vi "Open Recording File.vi"(8 "error in (no error)":errorcluster, 11 "IntanElectrophysiology in":refnum<class "IntanElectrophysiology.lvclass">) -> (0 "error out":errorcluster, 3 "IntanElectrophysiology out":refnum<class "IntanElectrophysiology.lvclass">)   [LabVIEW 2014, in "IntanElectrophysiology.lvclass"]
uses:
  IntanElectrophysiology.lvclass
  IntanElectrophysiology.lvclass/IntanElectrophysiology.ctl
  AcquireTraces/AcquireTraces.lvclass/AcquireTraces.ctl
  HDF5Tools/LabView/Create Dataset 2D Integer.vi
  HDF5Tools/LabView/HDF5Tools.lvlib
  AcquireTraces/AcquireTraces.lvclass
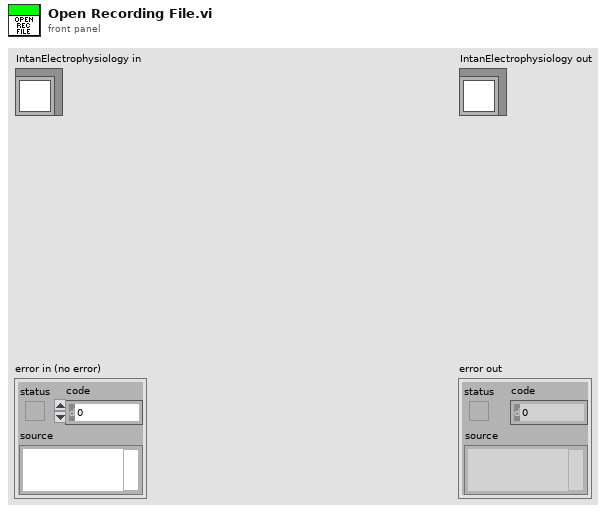
[diagram p1: front panel]
types:
  T1 = cluster{"Channels":string[], "SampClkRate":dbl, "AIDevScalingCoeff":dbl[], "Acq Channel Number":i32[], "Num Preamp Streams":i32, "Chans Per Preamp Stream":i32, "Num Board Channels":i32, "Samples Per Pkt Per Chan":i32}
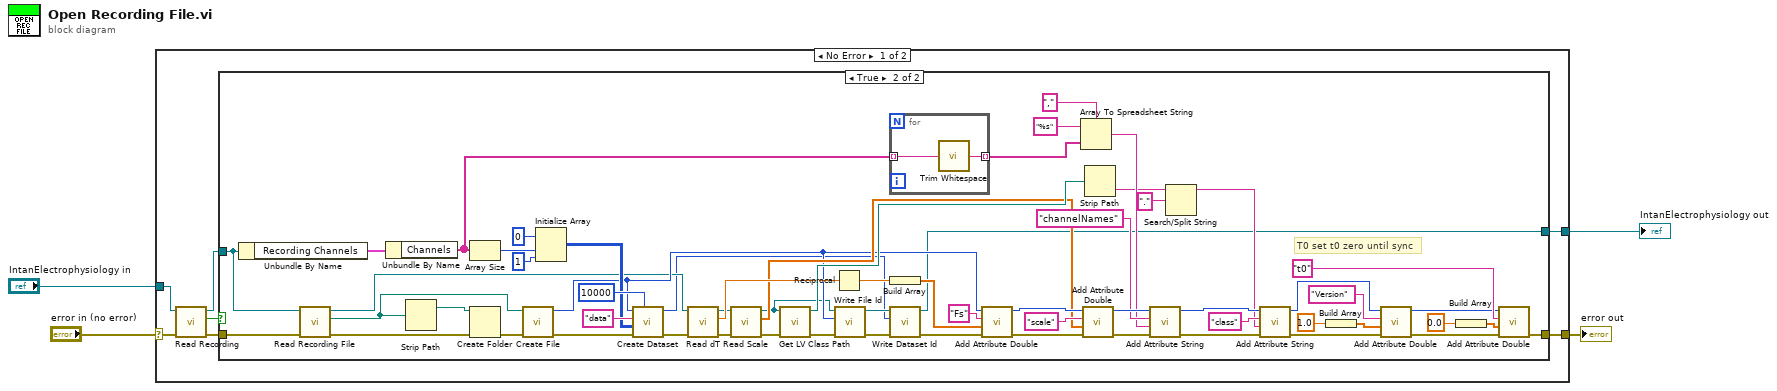
[diagram p0: block diagram]
diagram:
  n1 = case shown="No Error" "error in (no error)" {
    selector: "error in (no error)" -> [w6 w78]
    tunnel: [w10 w78] -> w1
    tunnel: [w11 w77] -> w2
    tunnel: "IntanElectrophysiology in" -> [w9 w77]
    frame No Error {
      n2 = call-dynamic "Read Recording.vi"("error in (no error)"=w6, "AcquireTraces in"=w9) -> ("error out"=w5:errorcluster, "Recording"=w7:bool, "AcquireTraces out"=w8:refnum<class "IntanElectrophysiology.lvclass">)  [unwired: 7 in]
      n3 = case shown="True" w7 {
        tunnel: w8 -> [w13 w68]
        tunnel: w5 -> [w12 w32]
        tunnel: [w13 w14] -> w11
        tunnel: [w12 w37] -> w10
        frame False {
        }
        frame True {
          # "T0 set t0 zero until sync"
          n4 = Unbundle By Name(w68) -> ("Recording Channels"=w26:T1)
          n5 = call-dynamic "Read Recording File.vi"("error in (no error)"=w32, "AcquistionObject in"=w68) -> ("error out"=w18:errorcluster, "Recording File"=w34:path, "AcquistionObject out"=w23:refnum<class "IntanElectrophysiology.lvclass">)  [unwired: 7 in]
          n6 = Unbundle By Name(w26) -> ("Channels"=w25:string[])
          n7 = Strip Path(path=w34) -> (stripped path=w35:path)  [unwired: 1 out]
          n8 = Array Size(array=w25) -> (size(s)=w55:i32)
          n9 = Create Folder(path (use dialog)=w35, error in=w18) -> (error out=w33:errorcluster)  [unwired: 1 in, 2 out]
          n10 = call "Create File.vi"("Error in"=w33, "File Name"=w34) -> ("Error out"=w74:errorcluster, "file_id"=w24:i32)  [unwired: 6 in]
          n11 = Initialize Array(0, w55, 1 ("dimension size")) -> (w69:i32[][])
          n12 = call-poly "Create Dataset.vi"("Chunk size"=10000, "error in (no error)"=w74, "Datatype"=w69, "Dataset name"="data", "Location id in"=w24) -> ("error out"=w17:errorcluster, "Dataset id"=w19:i32)  [unwired: 5 in]
          n13 = call-dynamic "Read dT.vi"("error in (no error)"=w17, "AcquireTraces in"=w23) -> ("error out"=w28:errorcluster, "dT"=w31:dbl, "AcquireTraces out"=w29:refnum<class "IntanElectrophysiology.lvclass">)  [unwired: 7 in]
          n14 = call-dynamic "Read Scale.vi"("error in (no error)"=w28, "AcquireTraces in"=w29) -> ("error out"=w27:errorcluster, "Scale (V/LSB)"=w30:dbl[], "AcquireTraces out"=w15:refnum<class "IntanElectrophysiology.lvclass">)  [unwired: 7 in]
          n15 = call <vilib>:"Get LV Class Path.vi"("error in (no error)"=w27, "object"=w15) -> ("error out"=w21:errorcluster, "class path"=w53:path)  [unwired: 8 in]
          n16 = Reciprocal(x=w31) -> (1/x=w42:dbl)
          n17 = call "Write File Id.vi"("error in (no error)"=w21, "File Id"=w24, "AcquireTraces in"=w15) -> ("error out"=w20:errorcluster, "AcquireTraces out"=w22:refnum<class "IntanElectrophysiology.lvclass">)  [unwired: 7 in]
          n18 = for {
            tunnel: w25 -> [w75] mode=indexing
            tunnel: [w76] -> w61 mode=indexing
            n19 = call <vilib>:"Trim Whitespace.vi"("string"=w75) -> ("trimmed string"=w76:string)  [unwired: 1 in]
          }
          n20 = Build Array(w42) -> (w66:dbl[])
          n21 = call "Write Dataset Id.vi"("error in (no error)"=w20, "Dataset Id"=w19, "AcquireTraces in"=w22) -> ("error out"=w16:errorcluster, "AcquireTraces out"=w14:refnum<class "IntanElectrophysiology.lvclass">)  [unwired: 7 in]
          n22 = call "Add Attribute Double.vi"("error in (no error)"=w16, "data"=w66, "Attribute name"="Fs", "loc_id"=w24) -> ("error out"=w65:errorcluster, "loc_id_out"=w58:i32)  [unwired: 6 in]
          n23 = Array To Spreadsheet String(delimiter (Tab)=",", array=w61, 3:"%s" ("format string")) -> (spreadsheet string=w56:string)
          n24 = call "Add Attribute Double.vi"("error in (no error)"=w65, "data"=w30, "Attribute name"="scale", "loc_id"=w58) -> ("error out"=w60:errorcluster, "loc_id_out"=w59:i32)  [unwired: 6 in]
          n25 = Strip Path(path=w53) -> (name=w52:string)  [unwired: 1 out]
          n26 = call "Add Attribute String.vi"("error in (no error)"=w60, "Attribute data"=w56, "Attribute name"="channelNames", "loc_id"=w59) -> ("error out"=w49:errorcluster, "loc_id_out"=w54:i32)  [unwired: 6 in]
          n27 = Search/Split String(string=w52, search string/char (-)=".") -> (substring before match=w48:string)  [unwired: 1 in, 2 out]
          n28 = call "Add Attribute String.vi"("error in (no error)"=w49, "Attribute data"=w48, "Attribute name"="class", "loc_id"=w54) -> ("error out"=w45:errorcluster, "loc_id_out"=w43:i32)  [unwired: 6 in]
          n29 = Build Array(1.0) -> (w44:dbl[])
          n30 = call "Add Attribute Double.vi"("error in (no error)"=w45, "data"=w44, "Attribute name"="Version", "loc_id"=w43) -> ("error out"=w39:errorcluster, "loc_id_out"=w38:i32)  [unwired: 6 in]
          n31 = Build Array(0.0 ("element")) -> (w40:dbl[])
          n32 = call "Add Attribute Double.vi"("error in (no error)"=w39, "data"=w40, "Attribute name"="t0", "loc_id"=w38) -> ("error out"=w37:errorcluster)  [unwired: 6 in, 1 out]
        }
      }
    }
    frame Error {
    }
  }
  "error out" <- w1
  "IntanElectrophysiology out" <- w2
